vi "Calculate stepsize for ramping.vi"(6 "TDAC voltages":dbl[](array[numeric]), 7 "Current step size":dbl, 8 "Loop iteration time":dbl, 9 "Previous set voltages":dbl[](array[numeric]), 10 "Set voltages":dbl[](array[numeric]), 11 "Ramp time":dbl) -> (3 "Step size":dbl)   [LabVIEW 2018]
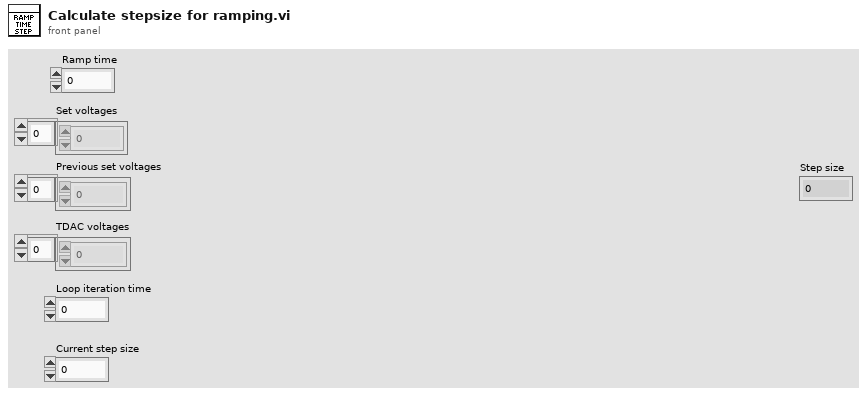
[diagram p1: front panel]
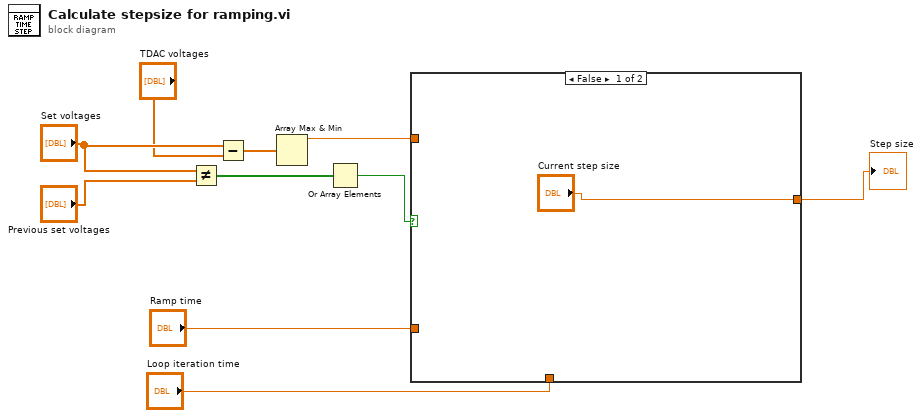
[diagram p0: block diagram]
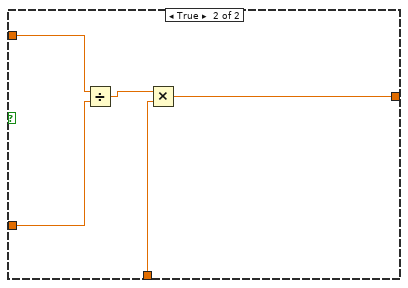
[diagram p2: hidden frame]
diagram:
  n1 = Not Equal?(x="Set voltages", y="Previous set voltages") -> (x != y?=w6:bool[])
  n2 = Subtract(x="Set voltages", y="TDAC voltages") -> (x-y=w8:dbl[])
  n3 = Array Max & Min(array=w8) -> (max value=w4:dbl)  [unwired: 3 out]
  n4 = Or Array Elements(Boolean array=w6) -> (logical OR=w5:bool)
  n5 = case shown="False" w5 {
    tunnel: w4 -> [_ w16]
    tunnel: "Ramp time" -> [_ w15]
    tunnel: "Loop iteration time" -> [_ w13]
    tunnel: ["Current step size" w12] -> w1
    frame False {
    }
    frame True {
      n6 = Divide(x=w16, y=w15) -> (x/y=w14:dbl)
      n7 = Multiply(x=w14, y=w13) -> (x*y=w12:dbl)
    }
  }
  "Step size" <- w1
